vi "Get Type Specializations Default.vi"(8 "error in":errorcluster) -> (0 "error out":errorcluster, 2 "parameter type specializations":T1[](array[typedef]))   [LabVIEW 2020, in "MeasurementServerTests.lvlib" / "Measurement Plugin Service Tests.lvlib"]
uses:
  Measurement Plugin Service Tests.lvlib
  Runtime/Measurements/Helpers/TypeDefs/Type Specialization.ctl
  Runtime/Measurements/Plug-In SDK Measurement.lvlib
  Runtime/Measurements/Helpers/TypeDefs/Type Specialization Key.ctl
  Runtime/Measurements/Helpers/TypeDefs/Parameter Type Specialization.ctl
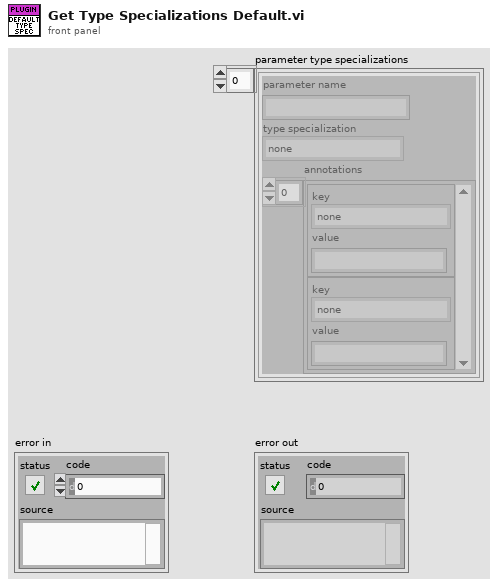
[diagram p1: front panel]
types:
  T1 = typedef "Plug-In SDK Measurement.lvlib/Parameter Type Specialization.ctl" = cluster{"parameter name":string, "type specialization":T2, "annotations":cluster{"key":T3, "value":string}[]}
  T2 = typedef "Plug-In SDK Measurement.lvlib/Type Specialization.ctl" = enum16{"none", "pin", "path", "enum", "ioresource"}
  T3 = typedef "Plug-In SDK Measurement.lvlib/Type Specialization Key.ctl" = enum16{"none", "pin.instrument_type", "enum.values", "ioresource.instrument_type"}
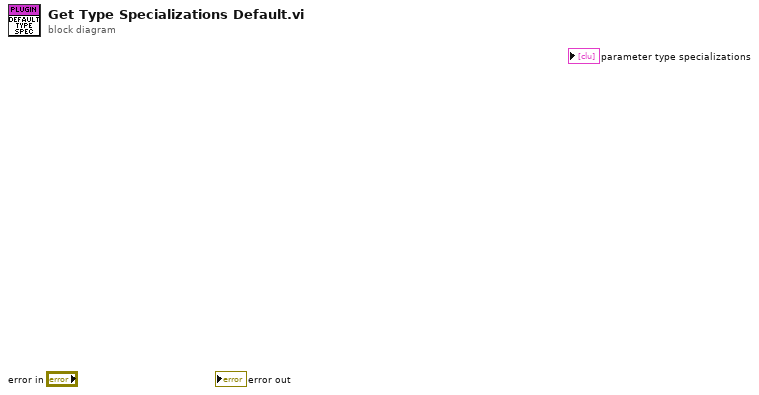
[diagram p0: block diagram]
diagram:
